vi "Get Transfer UIs.vi"(8 "error in (no error)":errorcluster, 11 "Component UI in":refnum<class "GE Reflective Memory User Interfaces.lvclass">) -> (0 "error out":errorcluster, 1 "Tx Transfer UI":refnum<class "User Interface.lvclass">, 2 "Rx Transfer UI":refnum<class "User Interface.lvclass">, 3 "Component UI out":refnum<class "GE Reflective Memory User Interfaces.lvclass">)   [LabVIEW 2020, in "GE Reflective Memory.lvlib" / "GE Reflective Memory User Interfaces.lvclass"]
uses:
  GE Reflective Memory User Interfaces.lvclass
  DSF Core.lvlibp/Classes/User Interface/User Interface.lvclass
  Transfer/Transfer User Interface.lvclass
  C:/Users/nitest/Desktop/Git 2020/niveristand-data-sharing-framework-custom-device-plugins/Components/DSF Core.lvlibp/Classes/User Interface/User Interface.lvclass
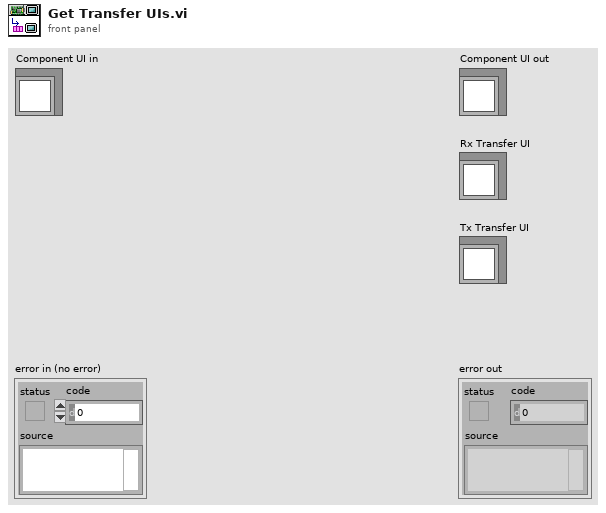
[diagram p1: front panel]
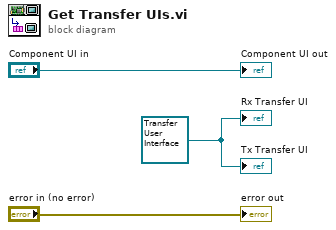
[diagram p0: block diagram]
diagram:
  w1 = refnum<class "Transfer User Interface.lvclass"> refnum ("GE Reflective Memory.lvlib:Transfer User Interface.lvclass")
  "error out" <- "error in (no error)"
  "Component UI out" <- "Component UI in"
  "Rx Transfer UI" <- w1
  "Tx Transfer UI" <- w1
